vi "Open Client Connection.vi"(8 "error in (no error)":errorcluster, 9 "Port":u16, 10 "address":string, 11 "RemoteControl.STM in":refnum<class "RemoteControl.STM.lvclass">) -> (0 "error out":errorcluster, 3 "RemoteControl.STM out":refnum<class "RemoteControl.STM.lvclass">)   [LabVIEW 2019, in "RemoteControl.STM.lvclass"]
uses:
  RemoteControl.STM.lvclass
  <vilib>/NI/STM/TCP/TCP Read Options.ctl
  RemoteControl.STM.lvclass/RemoteControl.STM.ctl
  <vilib>/NI/STM/TCP/Read Meta Data (TCP Ref).vi
  <vilib>/NI/STM/TCP/Read Meta Data (TCP Clst).vi
  <userlib>/LevyLab/RemoteControl/RemoteControl/RemoteControl.lvclass
  <vilib>/NI/STM/NI STM.lvlib
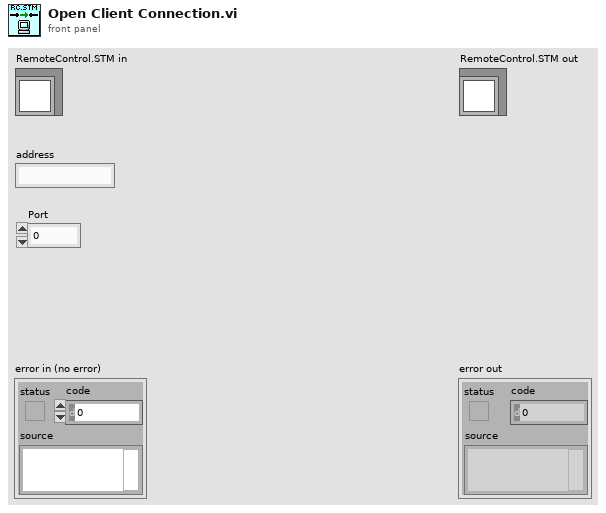
[diagram p1: front panel]
types:
  T1 = typedef "NI STM.lvlib/TCP Read Options.ctl" = cluster{"ignore timeout error":bool, "timeout ms (1000)":i32}
  T2 = typedef "NI STM.lvlib/TCP Connection Info.ctl" = cluster{"connection ID":refnum<k5>, "meta data":T3[]}
  T3 = typedef "NI STM.lvlib/MetaDataElement.ctl" = string
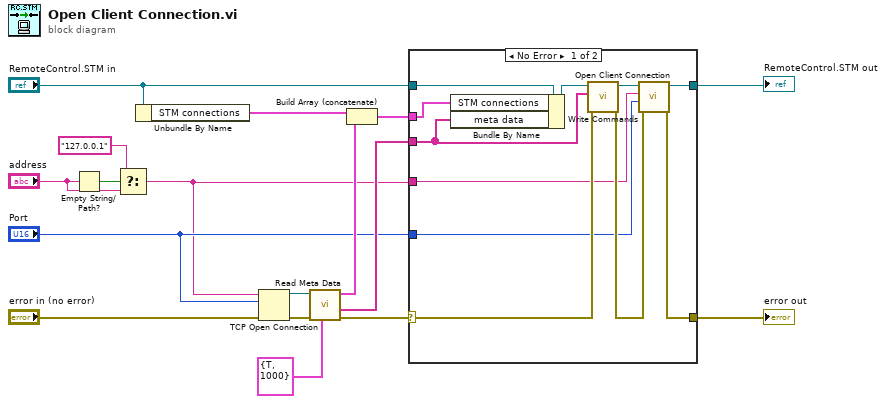
[diagram p0: block diagram]
diagram:
  n1 = Empty String/Path?(string/path="address") -> (empty?=w4:bool)
  n2 = Select(t="127.0.0.1", s=w4, f="address") -> (s? t:f=w1:string)
  n3 = Unbundle By Name("RemoteControl.STM in") -> ("STM connections"=w8:T2[])
  n4 = TCP Open Connection(address=w1, remote port or service name="Port", error in (no error)="error in (no error)") -> (connection ID=w16:refnum<k5>, error out=w17:errorcluster)  [unwired: 2 in]
  n5 = call-poly <vilib>:"Read Meta Data.vi"("options"=T1 {"ignore timeout error"=TRUE, "timeout ms (1000)"=1000}, "error in"=w17, "connection ID"=w16) -> ("error out"=w7:errorcluster, "meta data"=w11:T3[], "connection info out"=w15:T2)  [unwired: 6 in]
  n6 = Build Array (concatenate)(w8, w15) -> (w12:T2[])
  n7 = case shown="No Error" w7 {
    selector: w7 -> [w26 w30]
    tunnel: [w22 w30] -> w13
    tunnel: w12 -> [w18 _]
    tunnel: w11 -> [w21 _]
    tunnel: "RemoteControl.STM in" -> [w27 w29]
    tunnel: [w24 w29] -> w6
    tunnel: w1 -> [w20 _]
    tunnel: "Port" -> [w19 _]
    frame No Error {
      n8 = Bundle By Name(cluster=w27, "STM connections"=w18, "meta data"=w21) -> (w28:refnum<class "RemoteControl.STM.lvclass">)
      n9 = call-dynamic "Write Commands.vi"("error in (no error)"=w26, "Commands"=w21, "RemoteControl in"=w28) -> ("error out"=w23:errorcluster, "RemoteControl out"=w25:refnum<class "RemoteControl.STM.lvclass">)  [unwired: 7 in]
      n10 = call-parent "Open Client Connection.vi"("error in (no error)"=w23, "Port"=w19, "address"=w20, "RemoteControl in"=w25) -> ("error out"=w22:errorcluster, "RemoteControl out"=w24:refnum<class "RemoteControl.STM.lvclass">)  [unwired: 6 in]
    }
    frame Error {
    }
  }
  "error out" <- w13
  "RemoteControl.STM out" <- w6
